vi "Set Grid Mode.vi"(8 "error in (no error)":errorcluster, 10 "Grid Mode":T1, 11 "SCADA in":refnum<class "SCADA.lvclass">) -> (0 "error out":errorcluster, 3 "SCADA out":refnum<class "SCADA.lvclass">)   [LabVIEW 2015, in "SCADA Core.lvlib" / "SCADA.lvclass"]
uses:
  SCADA.lvclass
  Controls/Grid Mode.ctl
  SCADA.lvclass/SCADA.ctl
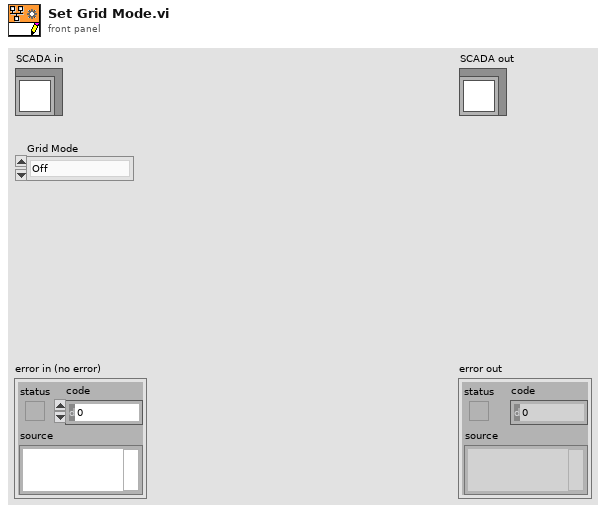
[diagram p1: front panel]
types:
  T1 = typedef "SCADA Core.lvlib/SCADA.lvclass/Grid Mode.ctl" = enum16{"Off", "Grid Connected", "Islanded", "Synchronizing"}
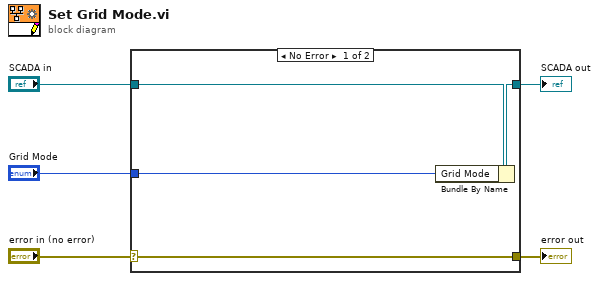
[diagram p0: block diagram]
diagram:
  n1 = case shown="No Error" "error in (no error)" {
    selector: "error in (no error)" -> [w9 w10]
    tunnel: [w9 w10] -> w4
    tunnel: [w7 w11] -> w2
    tunnel: "SCADA in" -> [w8 w11]
    tunnel: "Grid Mode" -> [w6 _]
    frame No Error {
      n2 = Bundle By Name(cluster=w8, "Grid Mode"=w6) -> (w7:refnum<class "SCADA.lvclass">)
    }
    frame Error {
    }
  }
  "error out" <- w4
  "SCADA out" <- w2
